vi "GetText.vi"(8 "error in":errorcluster, 11 "CVT editor node in":refnum<class "CVT editor node.lvclass">) -> (0 "error out":errorcluster, 1 "additional text":string, 2 "text":string, 3 "CVT editor node out":refnum<class "CVT editor node.lvclass">, 4 "glyph":string)   [LabVIEW 2013, in "CVT editor node.lvclass"]
uses:
  CVT editor node.lvclass
  <vilib>/NI/DCAF/Tag Editor Core/Configuration Editor/Classes/Module editor node/Read display name.vi
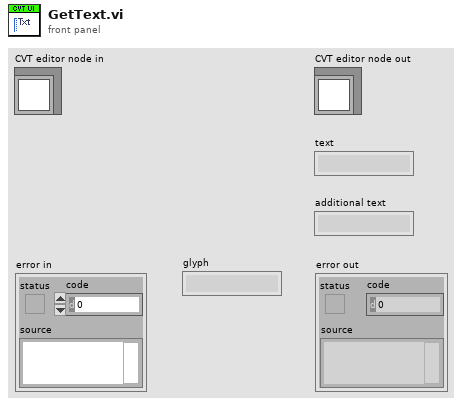
[diagram p1: front panel]
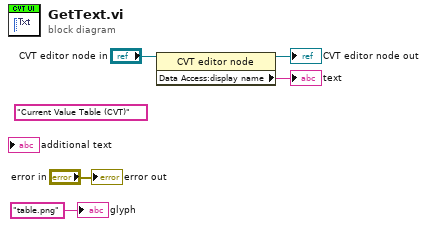
[diagram p0: block diagram]
diagram:
  (unwired) "Current Value Table (CVT)" ("text")
  n1 = property class="CVT editor node"(reference="CVT editor node in") -> (reference out=→"CVT editor node out":refnum<class "CVT editor node.lvclass">, "Data Access:display name"=→"text":string)  [unwired: 1 in, 1 out]
  "error out" <- "error in"
  "glyph" <- "table.png" ("glyph")
